vi "Video Diagnostics.vi"() -> (0 "error out":errorcluster, 3 "Voltage":dbl=0.003)   [LabVIEW 2013]
doc: "Performs diagnostics on the video card installed on the motherboard."
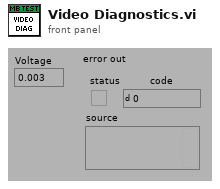
[diagram p1: front panel]
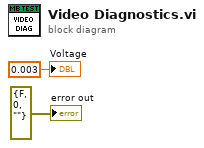
[diagram p0: block diagram]
diagram:
  "error out" <- errorcluster {"status"=FALSE, "code"=0, "source"=""} ("error out")
  "Voltage" <- 0.003 ("Numeric Measurement")
